vi "Start Sequence.vi"(8 "error in (no error)":errorcluster, 10 "Current Time":dbl, 11 "Output Sequencer in":refnum<class "Output Sequencer.lvclass">) -> (0 "error out":errorcluster, 2 "Sequencer State":T1, 3 "Output Sequencer out":refnum<class "Output Sequencer.lvclass">)   [LabVIEW 2020, in "Output Sequencer.lvlib" / "Output Sequencer.lvclass"]
uses:
  Output Sequencer.lvclass
  Types/Sequencer State.ctl
  Output Sequencer.lvclass/Output Sequencer.ctl
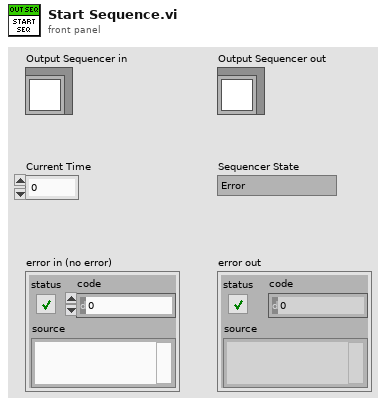
[diagram p1: front panel]
types:
  T1 = typedef "Output Sequencer.lvlib/Output Sequencer.lvclass/Sequencer State.ctl" = enum16{"Error", "Initialize", "Prepare channels", "Wait for test", "Wait for %.1f sec", "Wait for trigger", "Stop condition", "Wait for resume", "Running", "Paused", "No valid step", "Stopped"}
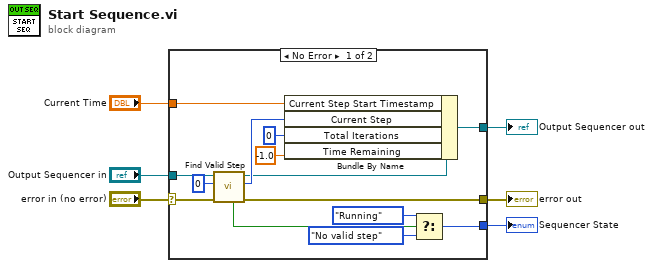
[diagram p0: block diagram]
diagram:
  n1 = case shown="No Error" "error in (no error)" {
    selector: "error in (no error)" -> [w11 w22]
    tunnel: [w20 w22] -> w6
    tunnel: "Current Time" -> [w17 _]
    tunnel: [w16 w21] -> w4
    tunnel: "Output Sequencer in" -> [w12 w21]
    tunnel: [w7 _] -> w2
    frame No Error {
      n2 = call "Find Valid Step.vi"("error in (no error)"=w11, "Starting Step"=0, "Output Sequencer in"=w12) -> ("error out"=w20:errorcluster, "Next Step"=w15:i32, "Output Sequencer out"=w13:refnum<class "Output Sequencer.lvclass">, "Valid Step Found"=w10:bool)  [unwired: 4 in, 1 out]
      n3 = Bundle By Name(cluster=w13, "Current Step Start Timestamp"=w17, "Current Step"=w15, "Total Iterations"=0 ("State.Total Iterations"), "Time Remaining"=-1.0 ("State.Time Remaining")) -> (w16:refnum<class "Output Sequencer.lvclass">)
      n4 = Select(t=Sequencer_State."Running" ("State.Sequencer State"), s=w10, f=Sequencer_State."No valid step" ("State.Sequencer State")) -> (s? t:f=w7:T1)
    }
    frame Error {
    }
  }
  "error out" <- w6
  "Output Sequencer out" <- w4
  "Sequencer State" <- w2
